vi "test.vi"() -> ()   [LabVIEW 2013]
panel:
  out "Numeric":u8
  in  "Boolean 2":bool
  in  "Boolean 1":bool
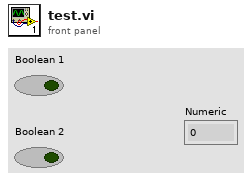
[diagram p1: front panel]
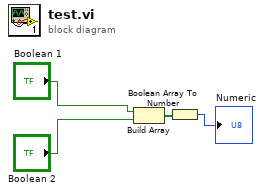
[diagram p0: block diagram]
diagram:
  n1 = Build Array("Boolean 1", "Boolean 2") -> (w4:bool[])
  n2 = Boolean Array To Number(Boolean array=w4) -> (number=→"Numeric":u8)
